vi "Sort_USNO_data.vi"(8 "Column Used":i32, 11 "Data IN":string[][](array[string])) -> (0 "n_elements":i32, 3 "Data OUT":string[][](array[string]))   [LabVIEW 2011]
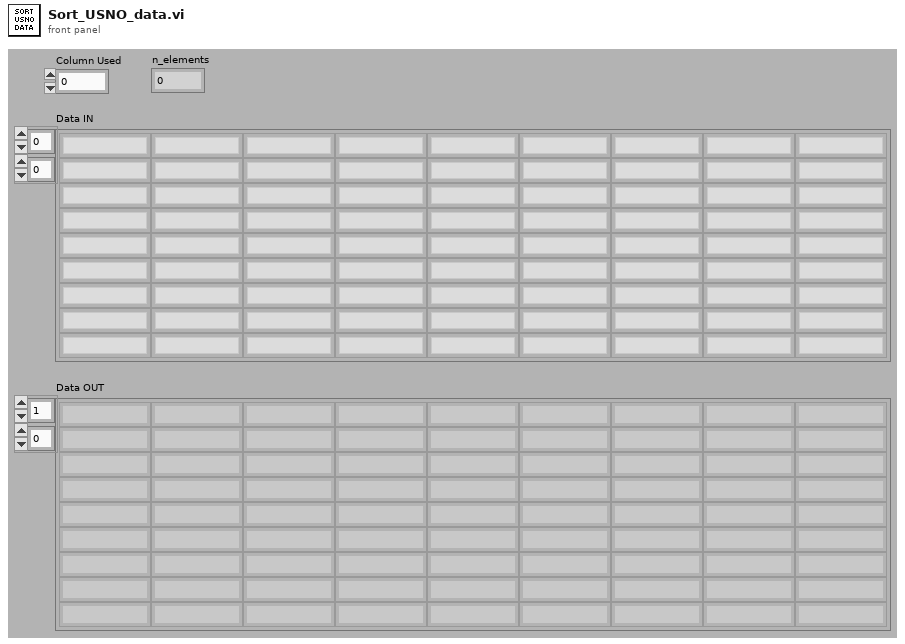
[diagram p1: front panel]
types:
  T1 = cluster{"String":string, "String":string, "String":string, "String":string, "String":string, "String":string, "String":string, "String":string, "String":string}[]
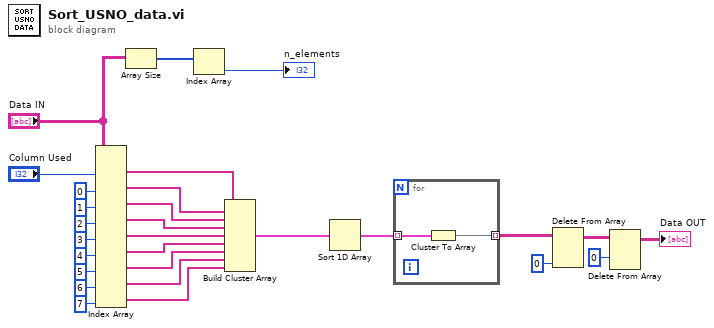
[diagram p0: block diagram]
diagram:
  n1 = Index Array(array="Data IN", index (col) #1="Column Used", index (col) #2=0 ("index (col)"), index (col) #3=1 ("index (col)"), index (col) #4=2 ("index (col)"), index (col) #5=3 ("index (col)"), index (col) #6=4 ("index (col)"), index (col) #7=5 ("index (col)"), index (col) #8=6 ("index (col)"), index (col) #9=7 ("index (col)")) -> (element #1=w7:string[], element #2=w19:string[], element #3=w18:string[], element #4=w17:string[], element #5=w16:string[], element #6=w15:string[], element #7=w14:string[], element #8=w13:string[], element #9=w12:string[])  [unwired: 9 in]
  n2 = Array Size(array="Data IN") -> (size(s)=w5:i32[])
  n3 = Index Array(array=w5) -> (element=→"n_elements":i32)  [unwired: 1 in]
  n4 = Build Cluster Array(w7, w19, w18, w17, w16, w15, w14, w13, w12) -> (w11:T1)
  n5 = Sort 1D Array(array=w11) -> (sorted array=w10:T1)
  n6 = for {
    tunnel: w10 -> [w30] mode=indexing
    tunnel: [w29] -> w9 mode=indexing
    n7 = Cluster To Array(cluster=w30) -> (array=w29:string[])
  }
  n8 = Delete From Array(array=w9, index (col)=0 ("disabled index (col)")) -> (array with subset deleted=w3:string[][])  [unwired: 2 in, 1 out]
  n9 = Delete From Array(array=w3, index (row)=0) -> (array with subset deleted=→"Data OUT":string[][])  [unwired: 2 in, 1 out]
